vi "Write HDF5.vi"(8 "error in (no error)":errorcluster, 9 "Cluster":T1, 10 "Filename":string, 11 "Path":path=path "C:/data") -> (0 "error out":errorcluster)   [LabVIEW 2009, in "Waveform.lvlib"]
uses:
  Waveform.lvlib
  interface/Dust Info.ctl
  interface/Timetrace.ctl
  interface/Data Source.ctl
  <vilib>/addons/_hdf5/property.llb/LVH5PClassId.ctl
  <vilib>/addons/_hdf5/property.llb/H5F_close_degree_t.ctl
  interface/Interface.lvlib
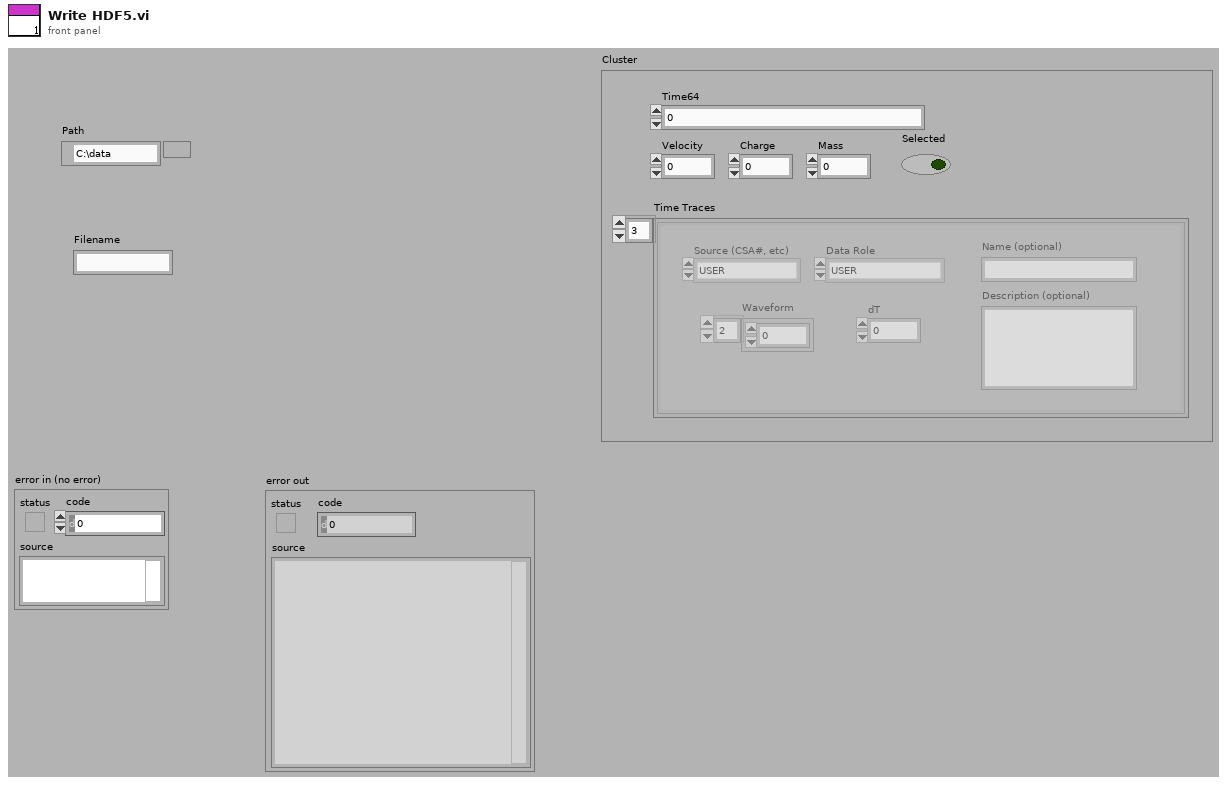
[diagram p1: front panel]
types:
  T1 = typedef "Interface.lvlib/Dust Info.ctl" = cluster{"Time64":u64, "Velocity":dbl, "Charge":dbl, "Mass":dbl, "Time Traces":T2[], "Selected":bool}
  T2 = typedef "Interface.lvlib/Timetrace.ctl" = cluster{"Source (CSA#, etc)":T3, "Data Role":enum16{"USER", "FIRST DETECTOR", "SECOND DETECTOR", "THIRD DETECTOR", "FINAL DETECTOR"}, "Waveform":sgl[], "dT":sgl, "Name (optional)":string, "Description (optional)":string}
  T3 = typedef "Interface.lvlib/Data Source.ctl" = enum16{"USER", "CSA1", "CSA2", "CSA3", "CSA4", "CSA5", "CSA6", ""}
  T4 = typedef "H5F_close_degree_t.ctl" = i32
  T5 = typedef "LVH5PClassId.ctl" = enum32{"H5P_FILE_CREATE", "H5P_FILE_ACCESS", "H5P_DATASET_CREATE", "H5P_DATASET_XFER", "H5P_MOUNT"}
  T6 = enum16{"open", "open or create", "create or replace", "create", "open (read only)"}
  T7 = typedef "HDF5 Ref.ctl" = refnum<k1>
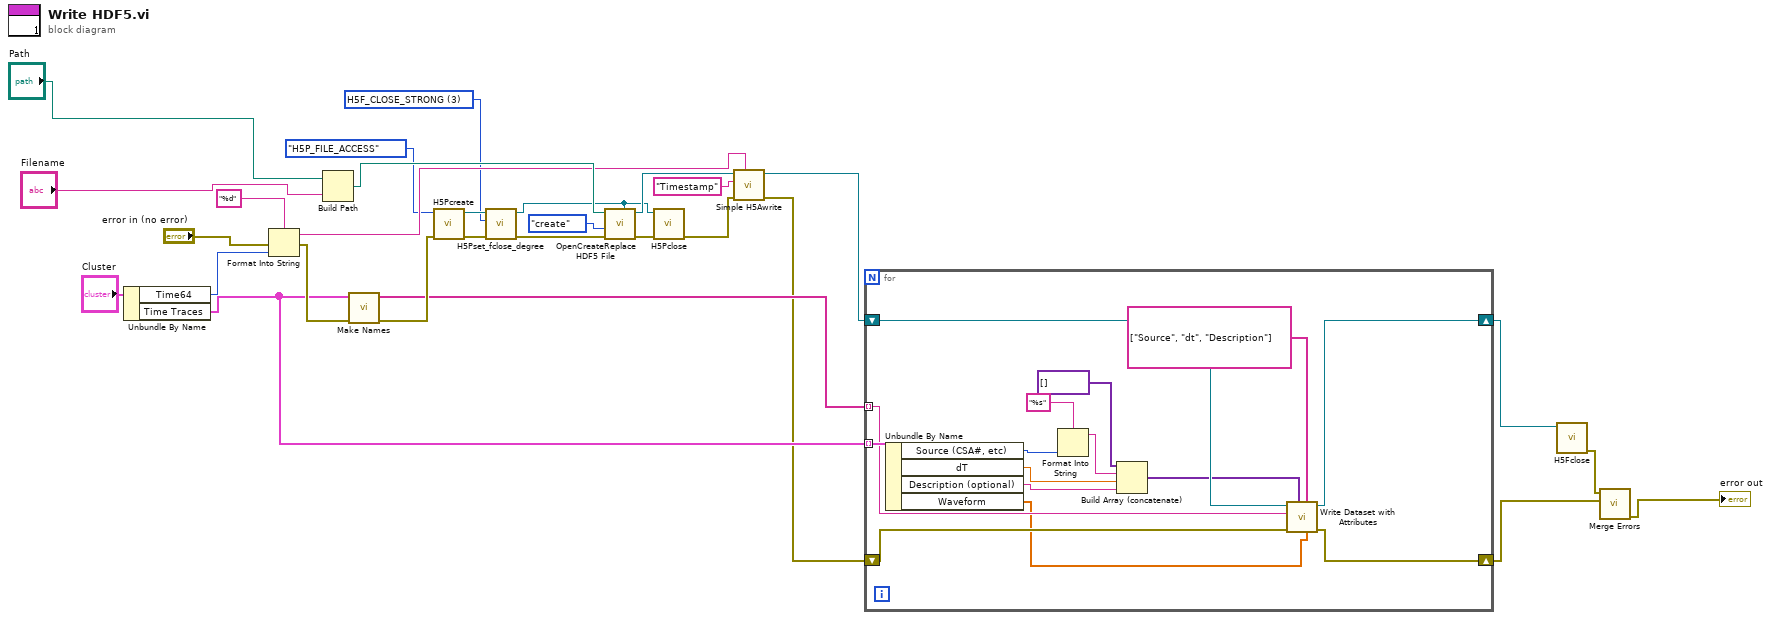
[diagram p0: block diagram]
diagram:
  w20 = T4 3 items=["H5F_CLOSE_DEFAULT", "H5F_CLOSE_WEAK", "H5F_CLOSE_SEMI", "H5F_CLOSE_STRONG"] ("Close degree")
  n1 = Unbundle By Name("Cluster") -> ("Time64"=w14:u64, "Time Traces"=w10:T2[])
  n2 = Format Into String(format string="%d", error in="error in (no error)", w14) -> (resulting string=w25:string, error out=w12:errorcluster)  [unwired: 1 in]
  n3 = Build Path(base path="Path", name or relative path="Filename") -> (appended path=w29:path)
  n4 = call "Make Names.vi"("error in (no error)"=w12, "Timetraces in"=w10) -> ("error out"=w11:errorcluster, "Names out"=w9:string[])  [unwired: 6 in]
  n5 = call <vilib>:"H5Pcreate.vi"("error in (no error)"=w11, "Property List Class"=LVH5PClassId."H5P_FILE_ACCESS") -> ("error out"=w22:errorcluster, "HDF5 Property List Ref"=w21:T7)  [unwired: 6 in]
  n6 = call <vilib>:"H5Pset_fclose_degree.vi"("error in (no error)"=w22, "Close degree"=w20, "HDF5 Property List Ref"=w21) -> ("error out"=w19:errorcluster, "HDF5 Property List Ref out"=w17:T7)  [unwired: 5 in]
  n7 = call <vilib>:"OpenCreateReplace HDF5 File.vi"("access_id"=w17, "error in (no error)"=w19, "function (open:0)"=T6."create", "path"=w29) -> ("error out"=w18:errorcluster, "HDF5 Ref out"=w27:T7)  [unwired: 4 in]
  n8 = call <vilib>:"H5Pclose.vi"("error in (no error)"=w18, "HDF5 Property Ref"=w17) -> ("error out"=w16:errorcluster)  [unwired: 7 in]
  n9 = call <vilib>:"Simple H5Awrite.vi"("Value"=w25, "error in (no error)"=w16, "Name"="Timestamp", "HDF5 Ref"=w27) -> ("error out"=w8:errorcluster, "HDF5 Ref out"=w4:T7)  [unwired: 4 in]
  n10 = for {
    tunnel: w10 -> [w44] mode=indexing
    tunnel: w9 -> [w33] mode=indexing
    shift-right: [w31] -> w5
    shift-left: w8 -> [w37]
    shift-right: [w30] -> w7
    shift-left: w4 -> [w36]
    n11 = Unbundle By Name(w44) -> ("Source (CSA#, etc)"=w43:T3, "dT"=w39:sgl, "Description (optional)"=w38:string, "Waveform"=w32:sgl[])
    n12 = Format Into String(format string="%s", w43) -> (resulting string=w40:string)  [unwired: 2 in, 1 out]
    n13 = Build Array (concatenate)(variant[] [], w40, w39, w38) -> (w34:variant[])
    n14 = call <vilib>:"Write Dataset with Attributes.vi"("Data"=w32, "Attribute Names"=string[] ["Source", "dt", "Description"], "Attribute Values"=w34, "error in (no error)"=w37, "Dataset name"=w33, "HDF5 Ref"=w36) -> ("error out"=w31:errorcluster, "HDF5 Ref out"=w30:T7)  [unwired: 4 in]
  }
  n15 = call <vilib>:"H5Fclose.vi"("HDF5 Ref"=w7) -> ("error out"=w6:errorcluster)  [unwired: 8 in]
  n16 = call <vilib>:"Merge Errors.vi"("error in 2 (no error)"=w5, "error in 1 (no error)"=w6) -> ("error out"=→"error out":errorcluster)  [unwired: 5 in]
